vi "svc_Convert Sort Indices to Unsort Indices.vi"(1 "sort indices":i32[](array[numeric])) -> (0 "unsort indices":i32[](array[numeric]))   [LabVIEW 2017]
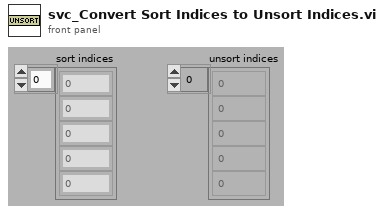
[diagram p1: front panel]
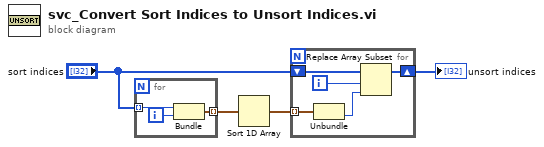
[diagram p0: block diagram]
diagram:
  n1 = for {
    tunnel: "sort indices" -> [w7] mode=indexing
    tunnel: [w6] -> w3 mode=indexing
    i -> [w5]
    n2 = Bundle(w7, w5) -> (w6:cluster{i32, i32})  [unwired: 1 in]
  }
  n3 = Sort 1D Array(array=w3) -> (sorted array=w4:cluster{i32, i32}[])
  n4 = for {
    tunnel: w4 -> [w12] mode=indexing
    shift-right: [w8] -> w1
    shift-left: "sort indices" -> [w11]
    i -> [w10]
    n5 = Unbundle(w12) -> (w9:i32)  [unwired: 1 out]
    n6 = Replace Array Subset(array=w11, new element=w9, index=w10) -> (w8:i32[])
  }
  "unsort indices" <- w1
